vi "LoadModel.vi"(8 "error in (no error)":errorcluster, 10 "Actor In":refnum<class "Actor.lvclass">, 11 "GRMActor in":refnum<class "MicroscopeController.lvclass">) -> (0 "error out":errorcluster, 3 "GRMActor out":refnum<class "MicroscopeController.lvclass">)   [LabVIEW 2020, in "MicroscopeController.lvlib" / "MicroscopeController.lvclass"]
uses:
  MicroscopeController.lvclass
  <vilib>/ActorFramework/Actor/Actor.lvclass
  Model/Hardware Layer/Real Hardware/Microscope_RM21/Microscope_RM21/Microscope_RM21.lvclass
  C:/Program Files/National Instruments/LabVIEW 2020/vi.lib/ActorFramework/Actor/Actor.lvclass
  MicroscopeController.lvclass/MicroscopeController.ctl
  Model/Hardware Abstraction Layer/Component/GenericActor/GenericActor/GenericController.lvclass
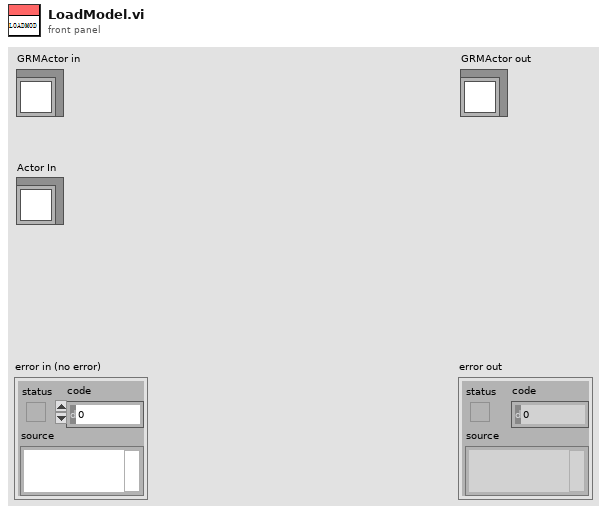
[diagram p1: front panel]
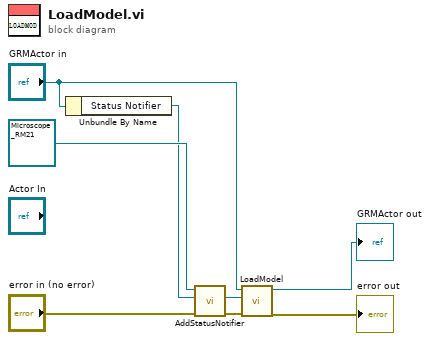
[diagram p0: block diagram]
diagram:
  n1 = Unbundle By Name("GRMActor in") -> ("Status Notifier"=w1:refnum<notifier>)
  n2 = call-dynamic "AddStatusNotifier.vi"("error in (no error)"="error in (no error)", "Status Notifier"=w1, "Microscope in"=refnum<class "Microscope_RM21.lvclass"> refnum ("Microscope_RM21.lvlib:Microscope_RM21.lvclass")) -> ("error out"=w5:errorcluster, "Microscope out"=w3:refnum<class "Microscope_RM21.lvclass">)  [unwired: 7 in]
  n3 = call-parent "LoadModel.vi"("error in (no error)"=w5, "Actor In"=w3, "GRMActor in"="GRMActor in") -> ("error out"=→"error out":errorcluster, "GRMActor out"=→"GRMActor out":refnum<class "MicroscopeController.lvclass">)  [unwired: 7 in]
